vi "Path Edit.vi"() -> ()   [LabVIEW 2019]
uses:
  Classes/Settings/ObjectSettings/ObjectSettings.lvclass/ObjectSettings.ctl
  Classes/Settings/Path Settings/Path Settings.lvclass/Path Settings.ctl
  typedefs/Schedule Types/Schedule--Constant.ctl
  Classes/Settings/Setting Database/Setting Database.lvclass
  Classes/Settings/Path Settings/Path Settings.lvclass
  C:/Users/Albro/Documents/GitHub/AFM-Lithography/lvsrc/Classes/Settings/ObjectSettings/ObjectSettings.lvclass
  Classes/Settings/Setting Database/Typedefs/PrivateEvents--Setting Database.SetDefaultPath.ctl
  <vilib>/JKI/JKI SMO/SMO/SMO.lvclass
  Classes/Settings/Setting Database/Typedefs/PrivateEvents--Setting Database.CopyActivePathToAll.ctl
  Classes/Settings/ObjectSettings/Accessors/Write Voltage Schedule.vi
  Classes/Settings/ObjectSettings/Accessors/Write Speed Schedule.vi
  Classes/Settings/ObjectSettings/Accessors/Write Direction.vi
  Classes/Settings/ObjectSettings/Accessors/Write Resistance.vi
  Classes/Settings/ObjectSettings/Accessors/Write Enabled.vi
  Classes/Settings/Path Settings/Accessors/Write Fill Orientation.vi
  Classes/Settings/Path Settings/Accessors/Write Smooth Segments.vi
  Classes/Settings/ObjectSettings/Accessors/Read Speed Settings.vi
  Classes/Settings/ObjectSettings/Accessors/Read Voltage Settings.vi
  Classes/Settings/Path Settings/Accessors/Write Fill Spacing.vi
  Classes/Settings/Path Settings/Accessors/Write Interpolation.vi
  Classes/Settings/Path Settings/Accessors/Read Interpolation.vi
  Classes/Settings/ObjectSettings/Accessors/Read Enabled.vi
  Classes/Settings/ObjectSettings/Accessors/Read Direction.vi
  Classes/Settings/Path Settings/Accessors/Read Fill Orientation.vi
  Classes/Settings/Path Settings/Accessors/Read Smooth Segments.vi
  Classes/Settings/Path Settings/Accessors/Read Fill Spacing.vi
  Classes/Settings/ObjectSettings/Accessors/Read Speed Schedule.vi
  Classes/Settings/ObjectSettings/Accessors/Read Voltage Schedule.vi
  Classes/Settings/ObjectSettings/Accessors/Read Resistance.vi
  Classes/Settings/ObjectSettings/ObjectSettings.lvclass
panel:
  out "ID String":string
  in  "Apply All":bool
  in  "Apply":bool
  out "Group String":string
  in  "Deviate Settings":bool
  in  "Deviate?":bool=TRUE
  in  "Save Default":bool
  in  "Interpolation":dbl caption="Numeric 2"
  in  "Voltage Settings":bool
  in  "Speed Settings":bool
  in  "Fill Spacing":dbl caption="Numeric 2"
  in  "Fill Orientation":u16(ring) caption="Ring" items=["Horizontal", "Vertical"]
  in  "Smooth Segments":dbl caption="Numeric 2"
  in  "Set Resistance":T1(ring) caption="Enum"
  in  "Copy to All":bool
  in  "Voltage (V)":dbl caption="Numeric 2"
  in  "Speed (um/s)":dbl caption="Numeric 2"
  in  "Voltage Schedule":u16(ring) caption="Ring" items=["Constant", "Ramp", "Fn. Generator", "Formula"]
  in  "Speed Schedule":u16(ring) caption="Ring" items=["Constant", "Ramp", "Fn. Generator", "Formula"]
  in  "Direction":u16(ring) caption="Ring" items=["Forward", "Backward"]
  in  "Enabled?":bool=TRUE
  in  "Index":i32=8
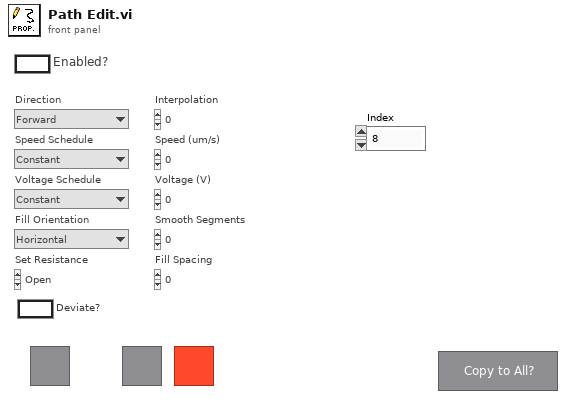
[diagram p1: front panel]
types:
  T1 = enum16{"Open", "Discharge Tip", "0 ohm", "100 kohm", "10 Mohm", "1 Gohm"}
  T2 = typedef "Schedule--Constant.ctl" = cluster{"Value":dbl}
  T3 = enum32{"invalid app kind", "Development System", "Run Time System", "Student Edition", "Embedded LabVIEW", "Evaluation", "Custom"}
  T4 = enum8{"Enabled", "Disabled", "Disabled and Grayed Out"}
  T5 = enum32{"Invalid", "Standard", "Closed", "Hidden", "Minimized", "Maximized"}
  T6 = typedef "Setting Database.lvclass/PrivateEvents--Setting Database.SetDefaultPath.ctl" = bool
  T7 = typedef "Setting Database.lvclass/PrivateEvents--Setting Database.CopyActivePathToAll.ctl" = bool
  T8 = typedef "Setting Database.lvclass/PublicEvents--Setting Database.NewActivePath.ctl" = refnum<class "Path Settings.lvclass">
  T9 = cluster{"Core":cluster{"Current VI Reference":refnum<vi>, "Close Panel on Exit?":bool}, "SettingDB":refnum<class "Setting Database.lvclass">, "Path Settings":refnum<class "Path Settings.lvclass">}
  T10 = cluster{"Current VI Reference":refnum<vi>, "Close Panel on Exit?":bool}
  T11 = typedef "Setting Database.lvclass/PublicEvents--Cluster.ctl" = cluster{"NewActivePath":refnum<user-event>, "PathsUpdated":refnum<user-event>, "RectanglesUpdated":refnum<user-event>, "NewActiveRectangle":refnum<user-event>, "NewActiveFunnel":refnum<user-event>, "FunnelsUpdated":refnum<user-event>, "NewActiveDot":refnum<user-event>, "DotsUpdated":refnum<user-event>}
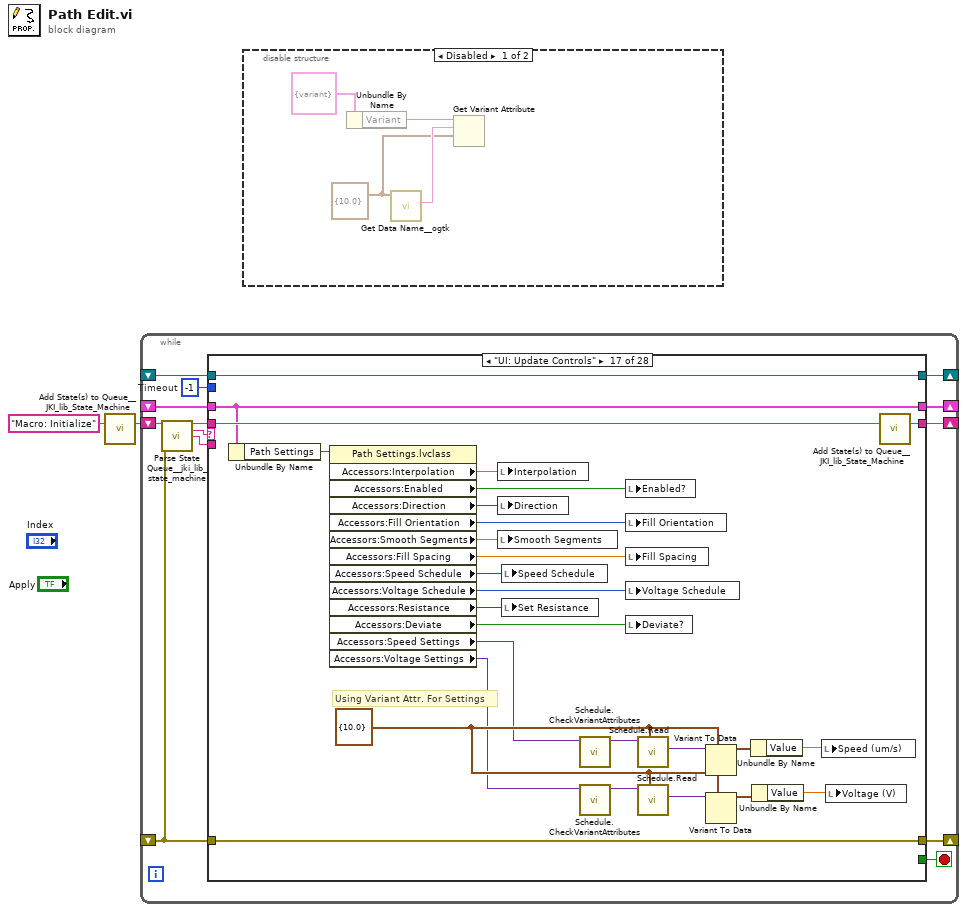
[diagram p0: block diagram]
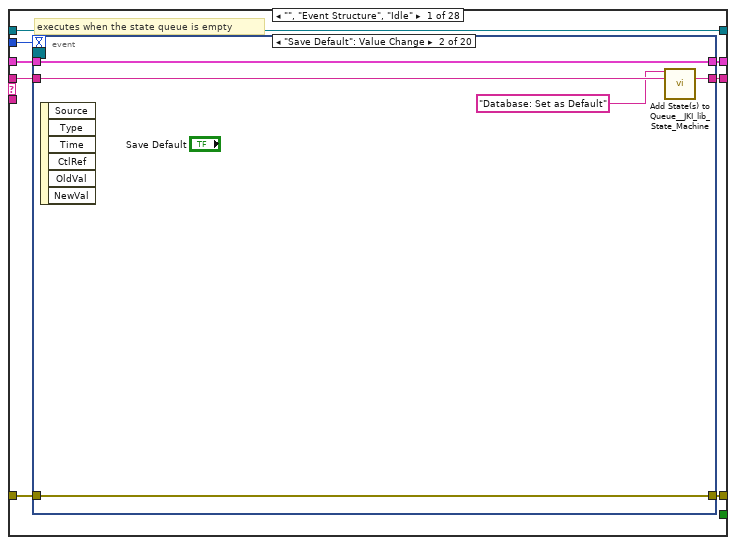
[diagram p3: hidden frame]
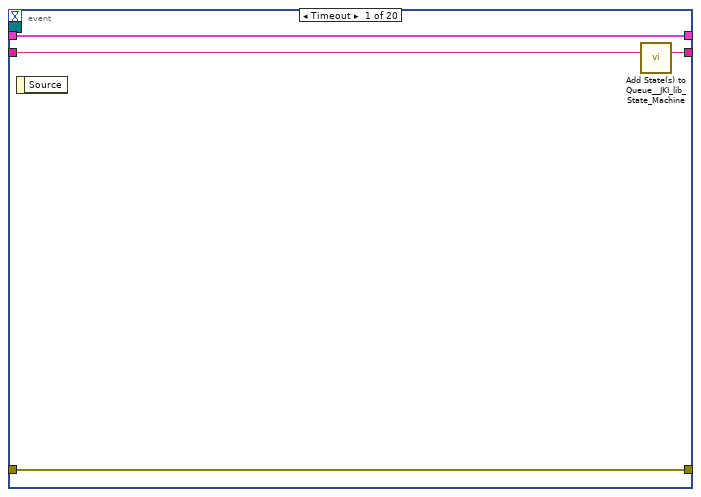
[diagram p4: hidden frame]
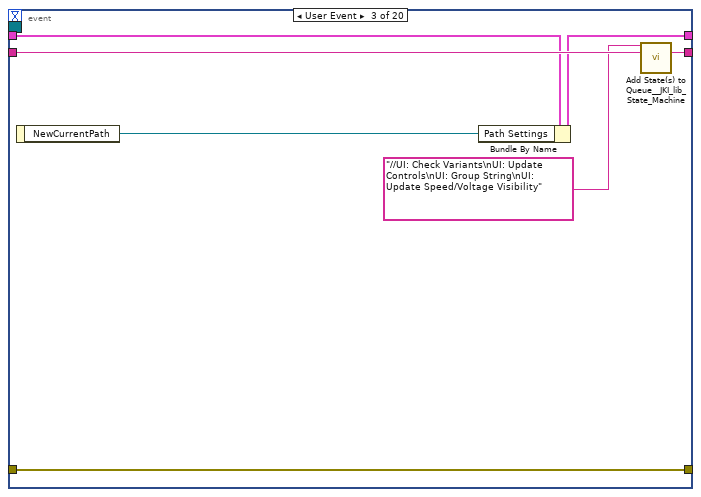
[diagram p5: hidden frame]
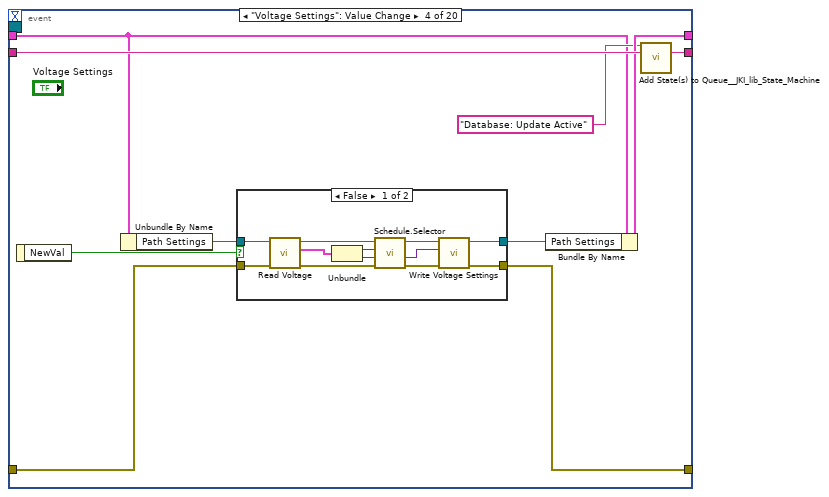
[diagram p6: hidden frame]
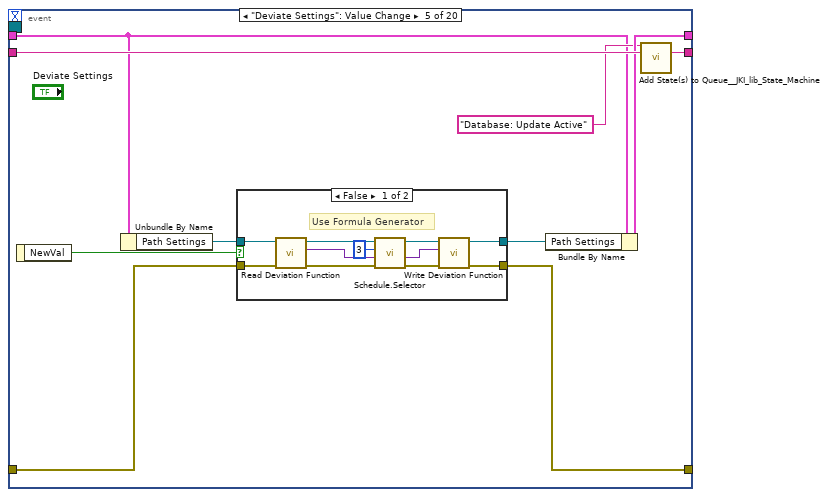
[diagram p8: hidden frame]
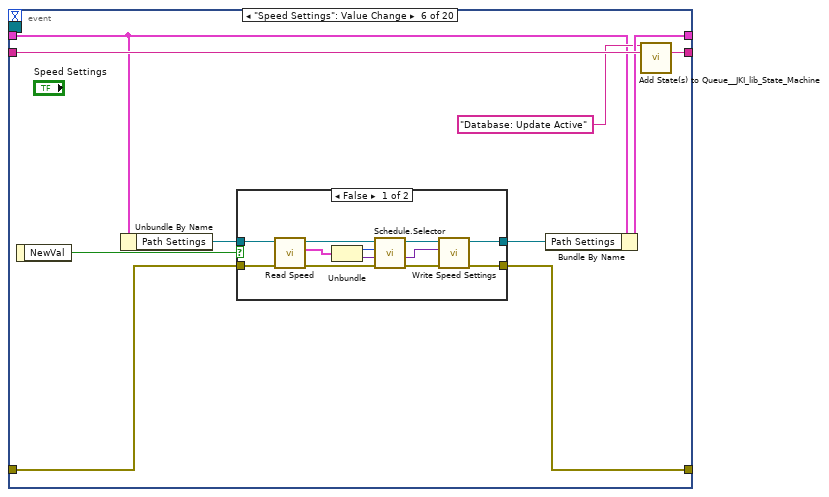
[diagram p10: hidden frame]
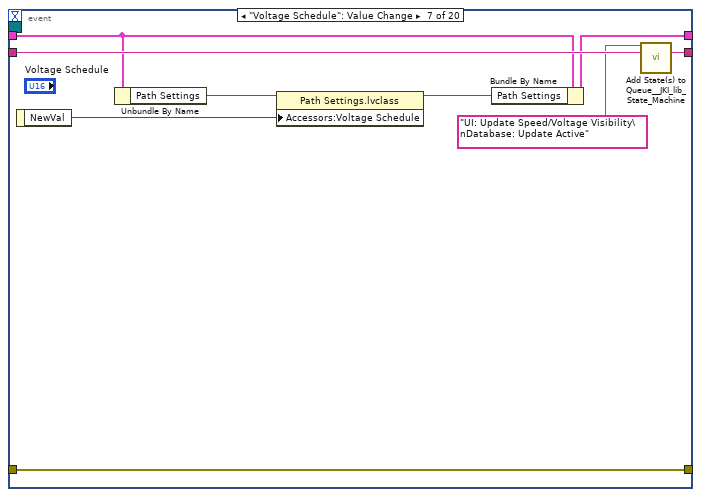
[diagram p12: hidden frame]
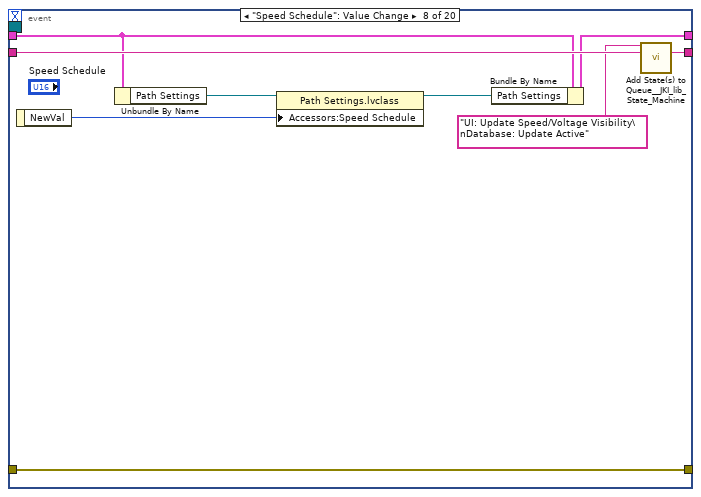
[diagram p13: hidden frame]
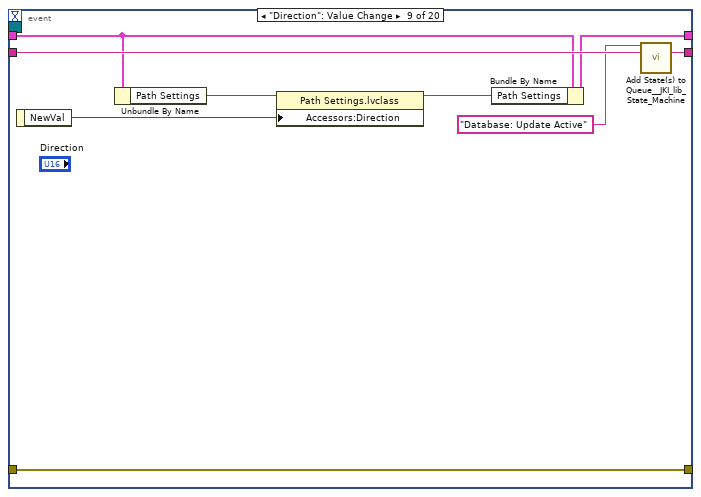
[diagram p14: hidden frame]
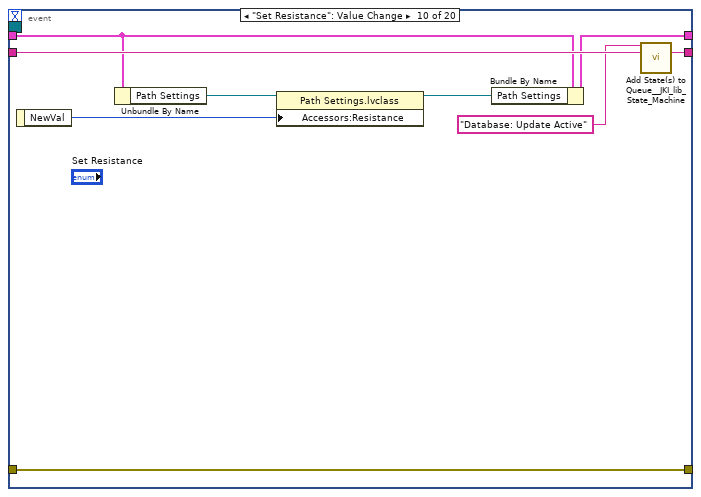
[diagram p15: hidden frame]
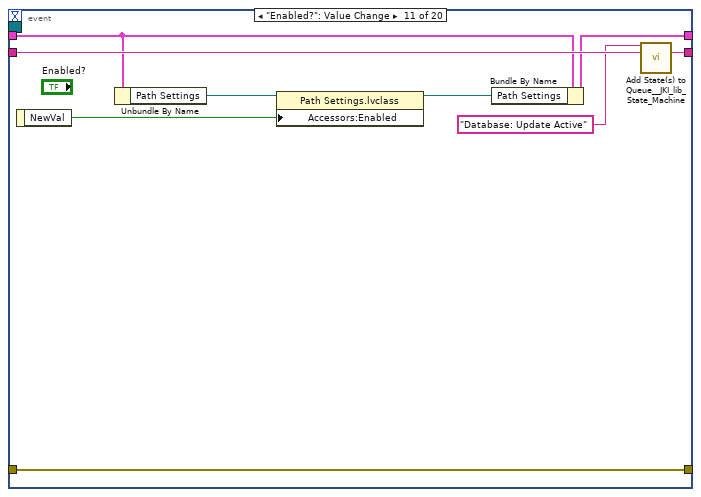
[diagram p16: hidden frame]
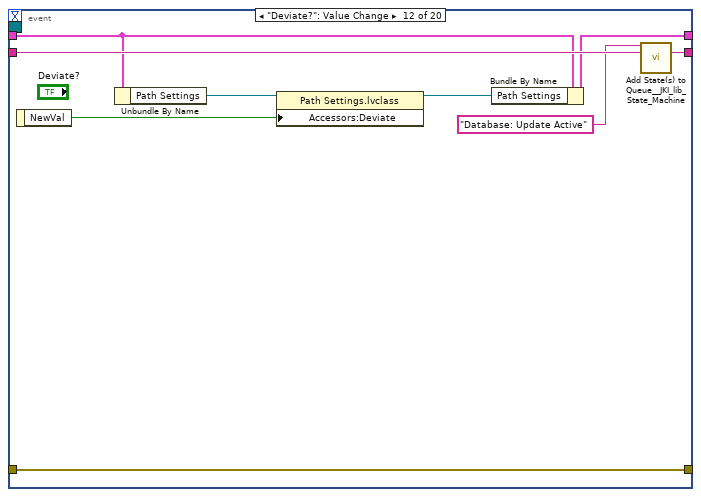
[diagram p17: hidden frame]
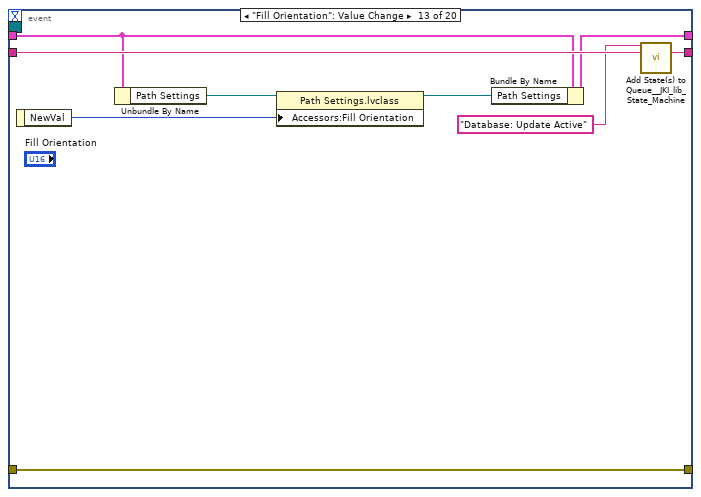
[diagram p18: hidden frame]
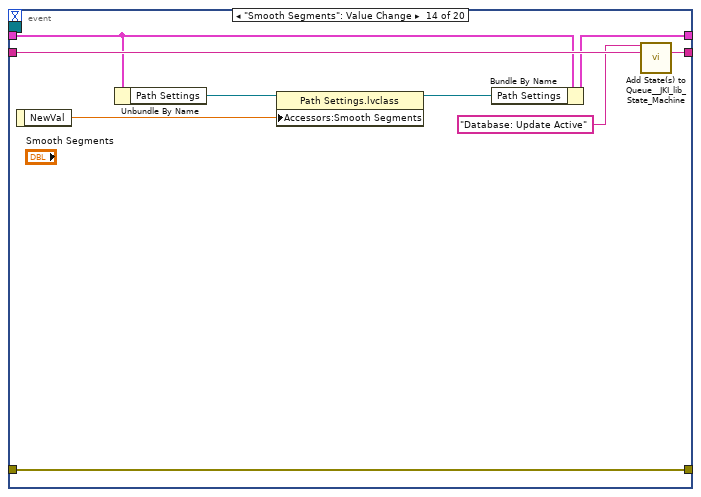
[diagram p19: hidden frame]
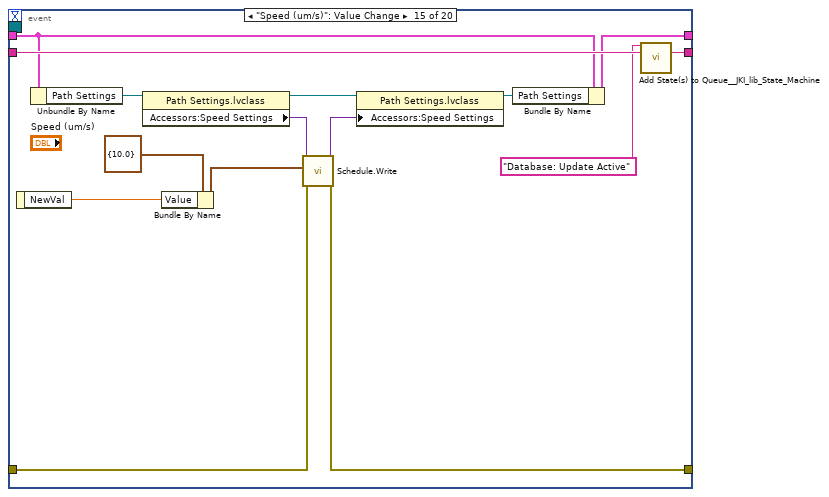
[diagram p20: hidden frame]
diagram:
  n1 = call <vilib>:"Add State(s) to Queue__JKI_lib_State_Machine.vi"("State(s) in (\"\")"="Macro: Initialize") -> ("States Out"=w2:string)  [unwired: 14 in]
  n2 = while "JKI - String-Based Queued State Machine (Basic) v1.0" {
    shift-right: [w8] -> _
    shift-left: _ -> [w6]
    shift-right: [w11] -> _
    shift-left: _ -> [w5]
    shift-right: [w10] -> _
    shift-left: w2 -> [w12]
    shift-right: [w4] -> _
    shift-left: _ -> [w3]
    stop <- w9 stop-if-true
    w7 = -1  # Timeout
    n3 = call <vilib>:"Parse State Queue__jki_lib_state_machine.vi"("State Queue"=w12, "Error In (no error)"=w5) -> ("Remaining States"=w14:string, "Current State"=w15:string, "Arguments"=w13:string)  [unwired: 11 in]
    n4 = case shown="\"UI: Update Controls\"" w15 {
      selector: w15 -> [_ _ w252 _ _ _ _ _ _ _ _ _ _ _ _ _ _ _ _ _ _ _ _ _ _ _ _ _]
      tunnel: w14 -> [w23 w246 w248 w271 w278 w284 w289 w297 w304 w309 w319 w325 w330 w343 w356 w367 w394 w401 w420 w432 w459 w465 w476 w481 w491 w508 w518 w528]
      tunnel: w13 -> [_ _ _ _ _ _ _ _ _ _ _ _ _ _ _ _ _ w397 _ w427 _ _ _ _ _ _ _ _]
      tunnel: [w20 w244 w255 w269 errorcluster {"status"=FALSE, "code"=0, "source"=""} ("error out") w282 w287 w294 w299 w307 w312 w320 w328 w333 w354 w358 w392 w398 w408 w429 w457 w463 w474 w479 w484 w506 w510 w520] -> w11
      tunnel: w5 -> [w19 w244 w254 w269 w275 w282 w287 w294 w300 w307 w310 w321 w328 w339 w354 w361 w392 w399 w416 w430 w457 w463 w474 w479 w483 w506 w509 w519]
      tunnel: [w22 w245 w253 w270 w277 w283 w288 w296 w303 w308 w318 w324 w329 w342 w355 w366 w393 w400 w419 w431 w458 w464 w475 w480 w490 w507 w517 w527] -> w10
      tunnel: [_ _ _ _ _ TRUE _ _ _ _ _ _ _ _ _ _ _ _ _ _ _ _ _ _ _ _ _ _] -> w9
      tunnel: [w18 w243 w251 w262 w273 w280 w286 w293 w301 w306 w316 w323 w327 w340 w352 w365 w388 w396 w418 w426 w456 w461 w468 w478 w488 w498 w515 w525] -> w8
      tunnel: w7 -> [w17 _ _ _ _ _ _ _ _ _ _ _ _ _ _ _ _ _ _ _ _ _ _ _ _ _ _ _]
      tunnel: w6 -> [w21 w243 w251 w263 w273 w280 w286 _ w301 w306 w316 w323 w327 w340 w351 w365 w388 w396 w418 w426 w456 w461 w468 w478 w487 w492 w514 w524]
      tunnel: [w16 w242 w247 w259 w272 w279 w285 w291 w298 w305 w317 w322 w326 w341 w353 w364 w389 w395 w406 w425 w455 w460 w466 w477 w489 w496 w516 w526] -> w4
      tunnel: w3 -> [w16 w242 w247 w259 w272 w279 w285 w291 w298 w305 _ w322 w326 w341 w353 w364 w389 w395 w406 w425 w455 w460 w466 w477 w489 w496 w516 w526]
      frame "", "Event Structure", "Idle" {
        # "executes when the state queue is empty"
        n5 = event shown="[1] \"Save Default\": Value Change" {
          selector: w16 -> [_ _ _ _ _ _ _ _ _ _ _ _ _ _ _ _ _ _ _ _]
          dyn-events: _ -> [_ _ _ _ _ _ _ _ _ _ _ _ _ _ _ _ _ _ _ _]
          timeout: w17 -> [_ _ _ _ _ _ _ _ _ _ _ _ _ _ _ _ _ _ _ _]
          tunnel: w23 -> [w27 w32 w39 w49 w73 w96 w119 w128 w137 w146 w155 w164 w173 w182 w197 w212 w221 w230 w235 w241]
          tunnel: [w26 w31 w38 w48 w72 w95 w118 w127 w136 w145 w154 w163 w172 w181 w196 w211 w220 w229 w234 w240] -> w22
          tunnel: w21 -> [w24 w29 w35 w45 w69 w92 w112 w121 w130 w139 w148 w157 w166 w175 w192 w207 w214 w223 w233 w238]
          tunnel: [w25 w30 w37 w41 w65 w88 w117 w126 w135 w144 w153 w162 w171 w180 w184 w199 w219 w228 w232 w239] -> w20
          tunnel: w19 -> [w25 w30 w37 w40 w64 w87 w117 w126 w135 w144 w153 w162 w171 w180 w183 w198 w219 w228 w232 w239]
          tunnel: [w24 w29 w36 w47 w71 w94 w116 w125 w134 w143 w152 w161 w170 w179 w195 w210 w218 w227 w233 w238] -> w18
          event Timeout {
            n6 = event-data() -> ()  [unwired: 1 in, 1 out]
            n7 = call <vilib>:"Add State(s) to Queue__JKI_lib_State_Machine.vi"("State(s) in (\"\")"=w27) -> ("States Out"=w26:string)  [unwired: 14 in]
          }
          event "Save Default": Value Change {
            n8 = event-data() -> ()  [unwired: 1 in, 6 out]
            n9 = call <vilib>:"Add State(s) to Queue__JKI_lib_State_Machine.vi"("State(s) in Front (\"\")"="Database: Set as Default", "State(s) in (\"\")"=w32) -> ("States Out"=w31:string)  [unwired: 13 in]
          }
          event User Event {
            n10 = event-data() -> ("NewCurrentPath"=w34:T8)  [unwired: 1 in]
            n11 = Bundle By Name(cluster=w35, "Path Settings"=w34) -> (w36:T9)
            n12 = call <vilib>:"Add State(s) to Queue__JKI_lib_State_Machine.vi"("State(s) in Front (\"\")"="//UI: Check Variants\nUI: Update Controls\nUI: Group String\nUI: Update Speed/Voltage Visibility", "State(s) in (\"\")"=w39) -> ("States Out"=w38:string)  [unwired: 13 in]
          }
          event "Voltage Settings": Value Change {
            n13 = event-data() -> ("NewVal"=w44:bool)  [unwired: 1 in]
            n14 = Unbundle By Name(w45) -> ("Path Settings"=w43:refnum<class "Path Settings.lvclass">)
            n15 = case shown="False" w44 {
              tunnel: w43 -> [w61 w63]
              tunnel: [w53 w63] -> w42
              tunnel: w40 -> [w60 w62]
              tunnel: [w50 w62] -> w41
              frame False {
                n16 = call "Read Voltage.vi"("error in (no error)"=w60, "ObjectSettings in"=w61) -> ("error out"=w58:errorcluster, "Voltage"=w57:cluster{"Schedule":u16, "Settings":variant}, "ObjectSettings out"=w59:refnum<class "Path Settings.lvclass">)  [unwired: 7 in]
                n17 = Unbundle(w57) -> ("Schedule"=w56:u16, "Settings"=w55:variant)
                n18 = call-dynamic "Schedule.Selector.vi"("error in (no error)"=w58, "Settings In"=w55, "Schedule"=w56, "ObjectSettings in"=w59) -> ("error out"=w52:errorcluster, "Settings Out"=w51:variant, "ObjectSettings out"=w54:refnum<class "Path Settings.lvclass">)  [unwired: 5 in]
                n19 = call "Write Voltage Settings.vi"("error in (no error)"=w52, "Settings"=w51, "ObjectSettings in"=w54) -> ("error out"=w50:errorcluster, "ObjectSettings out"=w53:refnum<class "Path Settings.lvclass">)  [unwired: 7 in]
              }
              frame True {
              }
            }
            n20 = Bundle By Name(cluster=w45, "Path Settings"=w42) -> (w47:T9)
            n21 = call <vilib>:"Add State(s) to Queue__JKI_lib_State_Machine.vi"("State(s) in Front (\"\")"="Database: Update Active", "State(s) in (\"\")"=w49) -> ("States Out"=w48:string)  [unwired: 13 in]
          }
          event "Deviate Settings": Value Change {
            n22 = event-data() -> ("NewVal"=w68:bool)  [unwired: 1 in]
            n23 = Unbundle By Name(w69) -> ("Path Settings"=w67:refnum<class "Path Settings.lvclass">)
            n24 = case shown="False" w68 {
              tunnel: w67 -> [w79 w86]
              tunnel: [w83 w86] -> w66
              tunnel: w64 -> [w76 w85]
              tunnel: [w80 w85] -> w65
              frame False {
                # "Use Formula Generator"
                n25 = call-dynamic "Read Deviation Function.vi"("error in (no error)"=w76, "Path Settings in"=w79) -> ("error out"=w77:errorcluster, "Deviation Function"=w75:variant, "Path Settings out"=w78:refnum<class "Path Settings.lvclass">)  [unwired: 7 in]
                n26 = call-dynamic "Schedule.Selector.vi"("error in (no error)"=w77, "Settings In"=w75, "Schedule"=u16 3, "ObjectSettings in"=w78) -> ("error out"=w82:errorcluster, "Settings Out"=w81:variant, "ObjectSettings out"=w84:refnum<class "Path Settings.lvclass">)  [unwired: 5 in]
                n27 = call-dynamic "Write Deviation Function.vi"("error in (no error)"=w82, "Deviation Function"=w81, "Path Settings in"=w84) -> ("error out"=w80:errorcluster, "Path Settings out"=w83:refnum<class "Path Settings.lvclass">)  [unwired: 7 in]
              }
              frame True {
              }
            }
            n28 = Bundle By Name(cluster=w69, "Path Settings"=w66) -> (w71:T9)
            n29 = call <vilib>:"Add State(s) to Queue__JKI_lib_State_Machine.vi"("State(s) in Front (\"\")"="Database: Update Active", "State(s) in (\"\")"=w73) -> ("States Out"=w72:string)  [unwired: 13 in]
          }
          event "Speed Settings": Value Change {
            n30 = event-data() -> ("NewVal"=w91:bool)  [unwired: 1 in]
            n31 = Unbundle By Name(w92) -> ("Path Settings"=w90:refnum<class "Path Settings.lvclass">)
            n32 = case shown="False" w91 {
              tunnel: w90 -> [w106 w110]
              tunnel: [w100 w110] -> w89
              tunnel: w87 -> [w104 w109]
              tunnel: [w99 w109] -> w88
              frame False {
                n33 = call "Read Speed.vi"("error in (no error)"=w104, "ObjectSettings in"=w106) -> ("error out"=w103:errorcluster, "Speed"=w102:cluster{"Schedule":u16, "Settings":variant}, "ObjectSettings out"=w105:refnum<class "Path Settings.lvclass">)  [unwired: 7 in]
                n34 = Unbundle(w102) -> ("Schedule"=w108:u16, "Settings"=w107:variant)
                n35 = call-dynamic "Schedule.Selector.vi"("error in (no error)"=w103, "Settings In"=w107, "Schedule"=w108, "ObjectSettings in"=w105) -> ("error out"=w98:errorcluster, "Settings Out"=w97:variant, "ObjectSettings out"=w101:refnum<class "Path Settings.lvclass">)  [unwired: 5 in]
                n36 = call "Write Speed Settings.vi"("error in (no error)"=w98, "Settings"=w97, "ObjectSettings in"=w101) -> ("error out"=w99:errorcluster, "ObjectSettings out"=w100:refnum<class "Path Settings.lvclass">)  [unwired: 7 in]
              }
              frame True {
              }
            }
            n37 = Bundle By Name(cluster=w92, "Path Settings"=w89) -> (w94:T9)
            n38 = call <vilib>:"Add State(s) to Queue__JKI_lib_State_Machine.vi"("State(s) in Front (\"\")"="Database: Update Active", "State(s) in (\"\")"=w96) -> ("States Out"=w95:string)  [unwired: 13 in]
          }
          event "Voltage Schedule": Value Change {
            n39 = event-data() -> ("NewVal"=w111:u16)  [unwired: 1 in]
            n40 = Unbundle By Name(w112) -> ("Path Settings"=w114:refnum<class "Path Settings.lvclass">)
            n41 = property class="Path Settings.lvclass"(reference=w114, "Accessors:Voltage Schedule"=w111) -> (reference out=w113:refnum<class "Path Settings.lvclass">)  [unwired: 1 in, 1 out]
            n42 = Bundle By Name(cluster=w112, "Path Settings"=w113) -> (w116:T9)
            n43 = call <vilib>:"Add State(s) to Queue__JKI_lib_State_Machine.vi"("State(s) in Front (\"\")"="UI: Update Speed/Voltage Visibility\nDatabase: Update Active", "State(s) in (\"\")"=w119) -> ("States Out"=w118:string)  [unwired: 13 in]
          }
          event "Speed Schedule": Value Change {
            n44 = event-data() -> ("NewVal"=w120:u16)  [unwired: 1 in]
            n45 = Unbundle By Name(w121) -> ("Path Settings"=w123:refnum<class "Path Settings.lvclass">)
            n46 = property class="Path Settings.lvclass"(reference=w123, "Accessors:Speed Schedule"=w120) -> (reference out=w122:refnum<class "Path Settings.lvclass">)  [unwired: 1 in, 1 out]
            n47 = Bundle By Name(cluster=w121, "Path Settings"=w122) -> (w125:T9)
            n48 = call <vilib>:"Add State(s) to Queue__JKI_lib_State_Machine.vi"("State(s) in Front (\"\")"="UI: Update Speed/Voltage Visibility\nDatabase: Update Active", "State(s) in (\"\")"=w128) -> ("States Out"=w127:string)  [unwired: 13 in]
          }
          event "Direction": Value Change {
            n49 = event-data() -> ("NewVal"=w129:u16)  [unwired: 1 in]
            n50 = Unbundle By Name(w130) -> ("Path Settings"=w132:refnum<class "Path Settings.lvclass">)
            n51 = property class="Path Settings.lvclass"(reference=w132, "Accessors:Direction"=w129) -> (reference out=w131:refnum<class "Path Settings.lvclass">)  [unwired: 1 in, 1 out]
            n52 = Bundle By Name(cluster=w130, "Path Settings"=w131) -> (w134:T9)
            n53 = call <vilib>:"Add State(s) to Queue__JKI_lib_State_Machine.vi"("State(s) in Front (\"\")"="Database: Update Active", "State(s) in (\"\")"=w137) -> ("States Out"=w136:string)  [unwired: 13 in]
          }
          event "Set Resistance": Value Change {
            n54 = event-data() -> ("NewVal"=w138:T1)  [unwired: 1 in]
            n55 = Unbundle By Name(w139) -> ("Path Settings"=w141:refnum<class "Path Settings.lvclass">)
            n56 = property class="Path Settings.lvclass"(reference=w141, "Accessors:Resistance"=w138) -> (reference out=w140:refnum<class "Path Settings.lvclass">)  [unwired: 1 in, 1 out]
            n57 = Bundle By Name(cluster=w139, "Path Settings"=w140) -> (w143:T9)
            n58 = call <vilib>:"Add State(s) to Queue__JKI_lib_State_Machine.vi"("State(s) in Front (\"\")"="Database: Update Active", "State(s) in (\"\")"=w146) -> ("States Out"=w145:string)  [unwired: 13 in]
          }
          event "Enabled?": Value Change {
            n59 = event-data() -> ("NewVal"=w147:bool)  [unwired: 1 in]
            n60 = Unbundle By Name(w148) -> ("Path Settings"=w150:refnum<class "Path Settings.lvclass">)
            n61 = property class="Path Settings.lvclass"(reference=w150, "Accessors:Enabled"=w147) -> (reference out=w149:refnum<class "Path Settings.lvclass">)  [unwired: 1 in, 1 out]
            n62 = Bundle By Name(cluster=w148, "Path Settings"=w149) -> (w152:T9)
            n63 = call <vilib>:"Add State(s) to Queue__JKI_lib_State_Machine.vi"("State(s) in Front (\"\")"="Database: Update Active", "State(s) in (\"\")"=w155) -> ("States Out"=w154:string)  [unwired: 13 in]
          }
          event "Deviate?": Value Change {
            n64 = event-data() -> ("NewVal"=w156:bool)  [unwired: 1 in]
            n65 = Unbundle By Name(w157) -> ("Path Settings"=w159:refnum<class "Path Settings.lvclass">)
            n66 = property class="Path Settings.lvclass"(reference=w159, "Accessors:Deviate"=w156) -> (reference out=w158:refnum<class "Path Settings.lvclass">)  [unwired: 1 in, 1 out]
            n67 = Bundle By Name(cluster=w157, "Path Settings"=w158) -> (w161:T9)
            n68 = call <vilib>:"Add State(s) to Queue__JKI_lib_State_Machine.vi"("State(s) in Front (\"\")"="Database: Update Active", "State(s) in (\"\")"=w164) -> ("States Out"=w163:string)  [unwired: 13 in]
          }
          event "Fill Orientation": Value Change {
            n69 = event-data() -> ("NewVal"=w165:u16)  [unwired: 1 in]
            n70 = Unbundle By Name(w166) -> ("Path Settings"=w168:refnum<class "Path Settings.lvclass">)
            n71 = property class="Path Settings.lvclass"(reference=w168, "Accessors:Fill Orientation"=w165) -> (reference out=w167:refnum<class "Path Settings.lvclass">)  [unwired: 1 in, 1 out]
            n72 = Bundle By Name(cluster=w166, "Path Settings"=w167) -> (w170:T9)
            n73 = call <vilib>:"Add State(s) to Queue__JKI_lib_State_Machine.vi"("State(s) in Front (\"\")"="Database: Update Active", "State(s) in (\"\")"=w173) -> ("States Out"=w172:string)  [unwired: 13 in]
          }
          event "Smooth Segments": Value Change {
            n74 = event-data() -> ("NewVal"=w174:dbl)  [unwired: 1 in]
            n75 = Unbundle By Name(w175) -> ("Path Settings"=w177:refnum<class "Path Settings.lvclass">)
            n76 = property class="Path Settings.lvclass"(reference=w177, "Accessors:Smooth Segments"=w174) -> (reference out=w176:refnum<class "Path Settings.lvclass">)  [unwired: 1 in, 1 out]
            n77 = Bundle By Name(cluster=w175, "Path Settings"=w176) -> (w179:T9)
            n78 = call <vilib>:"Add State(s) to Queue__JKI_lib_State_Machine.vi"("State(s) in Front (\"\")"="Database: Update Active", "State(s) in (\"\")"=w182) -> ("States Out"=w181:string)  [unwired: 13 in]
          }
          event "Speed (um/s)": Value Change {
            n79 = event-data() -> ("NewVal"=w190:dbl)  [unwired: 1 in]
            n80 = Unbundle By Name(w192) -> ("Path Settings"=w189:refnum<class "Path Settings.lvclass">)
            n81 = property class="Path Settings.lvclass"(reference=w189) -> (reference out=w188:refnum<class "Path Settings.lvclass">, "Accessors:Speed Settings"=w187:variant)  [unwired: 1 in, 1 out]
            n82 = Bundle By Name(cluster=T2 {"Value"=10.0} ("Constant"), "Value"=w190) -> (w185:T2)
            n83 = call "Schedule.Write.vi"("error in (no error)"=w183, "Data to Write"=w185, "LUT In"=w187) -> ("error out"=w184:errorcluster, "LUT Out"=w186:variant)  [unwired: 7 in]
            n84 = property class="Path Settings.lvclass"(reference=w188, "Accessors:Speed Settings"=w186) -> (reference out=w193:refnum<class "Path Settings.lvclass">)  [unwired: 1 in, 1 out]
            n85 = Bundle By Name(cluster=w192, "Path Settings"=w193) -> (w195:T9)
            n86 = call <vilib>:"Add State(s) to Queue__JKI_lib_State_Machine.vi"("State(s) in Front (\"\")"="Database: Update Active", "State(s) in (\"\")"=w197) -> ("States Out"=w196:string)  [unwired: 13 in]
          }
          event "Voltage (V)": Value Change {
            n87 = event-data() -> ("NewVal"=w205:dbl)  [unwired: 1 in]
            n88 = Unbundle By Name(w207) -> ("Path Settings"=w204:refnum<class "Path Settings.lvclass">)
            n89 = property class="Path Settings.lvclass"(reference=w204) -> (reference out=w203:refnum<class "Path Settings.lvclass">, "Accessors:Voltage Settings"=w202:variant)  [unwired: 1 in, 1 out]
            n90 = Bundle By Name(cluster=T2 {"Value"=10.0} ("Constant"), "Value"=w205) -> (w200:T2)
            n91 = call "Schedule.Write.vi"("error in (no error)"=w198, "Data to Write"=w200, "LUT In"=w202) -> ("error out"=w199:errorcluster, "LUT Out"=w201:variant)  [unwired: 7 in]
            n92 = property class="Path Settings.lvclass"(reference=w203, "Accessors:Voltage Settings"=w201) -> (reference out=w208:refnum<class "Path Settings.lvclass">)  [unwired: 1 in, 1 out]
            n93 = Bundle By Name(cluster=w207, "Path Settings"=w208) -> (w210:T9)
            n94 = call <vilib>:"Add State(s) to Queue__JKI_lib_State_Machine.vi"("State(s) in Front (\"\")"="Database: Update Active", "State(s) in (\"\")"=w212) -> ("States Out"=w211:string)  [unwired: 13 in]
          }
          event "Fill Spacing": Value Change {
            n95 = event-data() -> ("NewVal"=w213:dbl)  [unwired: 1 in]
            n96 = Unbundle By Name(w214) -> ("Path Settings"=w216:refnum<class "Path Settings.lvclass">)
            n97 = property class="Path Settings.lvclass"(reference=w216, "Accessors:Fill Spacing"=w213) -> (reference out=w215:refnum<class "Path Settings.lvclass">)  [unwired: 1 in, 1 out]
            n98 = Bundle By Name(cluster=w214, "Path Settings"=w215) -> (w218:T9)
            n99 = call <vilib>:"Add State(s) to Queue__JKI_lib_State_Machine.vi"("State(s) in Front (\"\")"="Database: Update Active", "State(s) in (\"\")"=w221) -> ("States Out"=w220:string)  [unwired: 13 in]
          }
          event "Interpolation": Value Change {
            n100 = event-data() -> ("NewVal"=w222:dbl)  [unwired: 1 in]
            n101 = Unbundle By Name(w223) -> ("Path Settings"=w225:refnum<class "Path Settings.lvclass">)
            n102 = property class="Path Settings.lvclass"(reference=w225, "Accessors:Interpolation"=w222) -> (reference out=w224:refnum<class "Path Settings.lvclass">)  [unwired: 1 in, 1 out]
            n103 = Bundle By Name(cluster=w223, "Path Settings"=w224) -> (w227:T9)
            n104 = call <vilib>:"Add State(s) to Queue__JKI_lib_State_Machine.vi"("State(s) in Front (\"\")"="Database: Update Active", "State(s) in (\"\")"=w230) -> ("States Out"=w229:string)  [unwired: 13 in]
          }
          event "Copy to All", "Apply All": Value Change {
            n105 = event-data() -> ()  [unwired: 1 in, 1 out]
            n106 = call <vilib>:"Add State(s) to Queue__JKI_lib_State_Machine.vi"("State(s) in Front (\"\")"="Database: Copy to All", "State(s) in (\"\")"=w235) -> ("States Out"=w234:string)  [unwired: 13 in]
          }
          event Panel Close? {
            # "Discard the event because we'll close the front panel ourselves in Macro: Exit"
            # "Close Panel button (pressed) Event\n(this executes Macro: Exit to terminate the VI)"
            n107 = event-data() -> ()  [unwired: 1 in, 1 out]
            n108 = event-data("Discard?"=TRUE) -> ()  [unwired: 1 in, 1 out]
            n109 = call <vilib>:"Add State(s) to Queue__JKI_lib_State_Machine.vi"("State(s) in Front (\"\")"="Macro: Exit", "State(s) in (\"\")"=w241) -> ("States Out"=w240:string)  [unwired: 13 in]
          }
        }
      }
      frame "---------- Core ----------" {
        # "Do not put any code in this frame.\n(it is a separator no-op)"
        n110 = call <vilib>:"Add State(s) to Queue__JKI_lib_State_Machine.vi"("State(s) in (\"\")"=w246) -> ("States Out"=w245:string)  [unwired: 14 in]
      }
      frame Default {
        w258 = 42 items=["No error", "Argument error", "Memory is full", "Out of zone", "End of file", "File already open", "Generic file I/O error", "File not found", "File permission error", "Disk is full", "Duplicate path", "Too many files open", "System feature not enabled", "Resource file not found", "Cannot add resource", "Resource not found", "Image not found", "Image memory error", "Pen does not exist", "Config type invalid", "Config token not found", "Config parse error", "Config memory error", "Bad external code format", "Bad external code offset", "External code not present", "Null window", "Destroy window error", "Null menu", "Print aborted", "Bad print record", "Print driver error", "Windows error during printing", "Memory error during printing", "Print dialog error", "Generic print error", "Invalid device refnum", "Device not found", "Device parameter error", "Device unit error", "Cannot open device", "Device call aborted", "Generic error", "Cancelled by user", "Object ID too low", "Object ID too high", "Object not in heap", "Unknown heap", "Unknown object (invalid DefProc)", "Unknown object (DefProc not in table)", "Message out of range", "Invalid (null) method", "Unknown message", "Manager call not supported", "Bad address", "Network operation in progress", "Network operation timed out", "Connection is busy", "Network attribute not supported", "Network error", "Address in use", "System out of memory", "Connection aborted", "Connection refused", "Not connected", "Already connected", "Connection closed", "Initialization error (interapplication manager)", "Bad occurrence", "Wait on unbound occurrence handler", "Occurrence queue overflow", "Datalog type conflict", "Unused", "Unrecognized type (interapplication manager)", "Memory corrupt", "Failed to make temporary DLL", "Old CIN version", "Drag socket not found", "Failed to load drop-object", "Failed to register OLE object", "Failed to release OLE object", "Format specifier type mismatch", "Unknown format specifier", "Too few format specifiers", "Too many format specifiers", "Scan failed", "Newer CIN version", "Error converting to variant", "Runtime menu error", "Password tampered", "Variant attribute not found", "Incompatible variant data type", "Event data is not available", "Event Store is not present", "Occurrence is not found", "Event Queue is not created", "Event info is not available", "Refnum passed is NULL", "Error retrieving Class GUID", "Error retrieving CoClass GUID", "Error retrieving TypeLib GUID.", "Bad built application magic bytes.", "Specific driver is different from the specific driver associated with the Logical Name.", "There is no session opened to the class driver.", "Max Error", "MAX - Error with config objects", "MAX - Error loading configuration", "MAX - Group not supported"]
        # "Current State"
        # "Do not delete, rename, or modify this frame.\n(this is used to capture unhandled states and typos)"
        # "Handle mistyped state name (developer tool)"
        n111 = Format Into String(format string="Software Exception: Unhandled State \"%s\"." ("message"), error in=w254, w252) -> (resulting string=w257:string, error out=w256:errorcluster)  [unwired: 1 in]
        n112 = call <vilib>:"Error Cluster From Error Code.vi"("show call chain? (False)"=TRUE, "error in (no error)"=w256, "error message (\"\")"=w257, "error code (0)"=w258) -> ("error out"=w255:errorcluster)  [unwired: 5 in]
        n113 = call <vilib>:"Add State(s) to Queue__JKI_lib_State_Machine.vi"("State(s) in (\"\")"=w248) -> ("States Out"=w253:string)  [unwired: 14 in]
      }
      frame "Initialize Core Data" {
        # "exe?"
        # "If panel starts closed or is an EXE, then close it when we exit"
        # "Do not delete, rename, or modify this frame.\n(this is used to determine panel behavior on exit)"
        n114 = control-ref of="Current VI Reference"() -> (w268:refnum<vi>)
        n115 = property class="VI"() -> ("Front Panel.Open"=w267:bool)  [unwired: 2 in, 2 out]
        n116 = property class="App"() -> ("App.Kind"=w266:T3)  [unwired: 2 in, 2 out]
        n117 = Not(x=w267) -> (.not. x?=w261:bool)
        n118 = Equal?(x=w266, y=T3."Run Time System" ("Application:Kind")) -> (x = y?=w260:bool)
        n119 = Or(x=w261, y=w260) -> (x .or. y?=w264:bool)
        n120 = Bundle By Name(cluster=w263, "Core.Current VI Reference"=w268, "Core.Close Panel on Exit?"=w264) -> (w262:T9)
        n121 = call <vilib>:"Add State(s) to Queue__JKI_lib_State_Machine.vi"("State(s) in (\"\")"=w271) -> ("States Out"=w270:string)  [unwired: 14 in]
      }
      frame "Error Handler" {
        # "Unhandled Error -- Display it"
        # "Handle any errors here.\nYou can also output any states to clean-up after errors occur"
        # "Clear error"
        n122 = call <vilib>:"General Error Handler.vi"("error in (no error)"=w275) -> ()  [unwired: 10 in, 5 out]
        n123 = call <vilib>:"Add State(s) to Queue__JKI_lib_State_Machine.vi"("State(s) in Front (\"\")"="/* Post Error States", "State(s) in (\"\")"=w278) -> ("States Out"=w277:string)  [unwired: 13 in]
      }
      frame "Exit" {
        # "Do not put any code in this frame.\n(No errors that occur here will be handled.)"
        n124 = call <vilib>:"Add State(s) to Queue__JKI_lib_State_Machine.vi"("State(s) in (\"\")"=w284) -> ("States Out"=w283:string)  [unwired: 14 in]
      }
      frame "---------- Data ----------" {
        # "Do not put any code in this frame.\n(It is a separator no-op. You can make a copy of this frame to create a new Data frame)"
        n125 = call <vilib>:"Add State(s) to Queue__JKI_lib_State_Machine.vi"("State(s) in (\"\")"=w289) -> ("States Out"=w288:string)  [unwired: 14 in]
      }
      frame "Data: Initialize" {
        w290 = refnum<class "Path Settings.lvclass"> refnum  # Path Settings
        w292 = refnum<class "Setting Database.lvclass"> refnum  # SettingDB
        w295 = T10 {"Current VI Reference"=refnum, "Close Panel on Exit?"=FALSE}  # Core
        # "Initialize the shift-register data, here.\n(data names are defined by what you wire into the bundle function)"
        n126 = Bundle("Core"=w295, "SettingDB"=w292, "Path Settings"=w290) -> (w293:T9)  [unwired: 1 in]
        n127 = call <vilib>:"Add State(s) to Queue__JKI_lib_State_Machine.vi"("State(s) in (\"\")"=w297) -> ("States Out"=w296:string)  [unwired: 14 in]
      }
      frame "Data: Cleanup" {
        # "Cleanup any data and references, here.\n(this is called automatically, by the Macro: Exit)"
        n128 = Unbundle By Name(w301) -> ("Core.Current VI Reference"=w302:refnum<vi>)
        n129 = Close Reference(reference=w302, error in (no error)=w300) -> (error out=w299:errorcluster)
        n130 = call <vilib>:"Add State(s) to Queue__JKI_lib_State_Machine.vi"("State(s) in (\"\")"=w304) -> ("States Out"=w303:string)  [unwired: 14 in]
      }
      frame "---------- Events ----------" {
        # "Do not put any code in this frame.\n(It is a separator no-op. You can make a copy of this frame to create a new UI frame)"
        n131 = call <vilib>:"Add State(s) to Queue__JKI_lib_State_Machine.vi"("State(s) in (\"\")"=w309) -> ("States Out"=w308:string)  [unwired: 14 in]
      }
      frame "Events: Register" {
        # "Do not put any code in this frame.\n(It is a separator no-op. You can make a copy of this frame to create a new UI frame)"
        n132 = Unbundle By Name(w316) -> ("SettingDB"=w315:refnum<class "Setting Database.lvclass">)
        n133 = call "Setting Database.GetPublicEvents.vi"("Setting Database"=w315) -> ("error out"=w311:errorcluster, "Public Events"=w314:T11)  [unwired: 8 in, 1 out]
        n134 = register-events(w314) -> (reference out=w317:refnum<event-registration>, error out=w313:errorcluster)  [unwired: 2 in]
        n135 = Merge Errors(w310, w313, w311) -> (w312:errorcluster)
        n136 = call <vilib>:"Add State(s) to Queue__JKI_lib_State_Machine.vi"("State(s) in (\"\")"=w319) -> ("States Out"=w318:string)  [unwired: 14 in]
      }
      frame "Events: Unregister" {
        # "Do not put any code in this frame.\n(It is a separator no-op. You can make a copy of this frame to create a new UI frame)"
        n137 = Unregister For Events(event registration refnum=w322, error in=w321) -> (error out=w320:errorcluster)
        n138 = call <vilib>:"Add State(s) to Queue__JKI_lib_State_Machine.vi"("State(s) in (\"\")"=w325) -> ("States Out"=w324:string)  [unwired: 14 in]
      }
      frame "---------- UI ----------" {
        # "Do not put any code in this frame.\n(It is a separator no-op. You can make a copy of this frame to create a new UI frame)"
        n139 = call <vilib>:"Add State(s) to Queue__JKI_lib_State_Machine.vi"("State(s) in (\"\")"=w330) -> ("States Out"=w329:string)  [unwired: 14 in]
      }
      frame "UI: Group String" {
        # "Do not put any code in this frame.\n(It is a separator no-op. You can make a copy of this frame to create a new UI frame)"
        n140 = Unbundle By Name(w340) -> ("Path Settings"=w332:refnum<class "Path Settings.lvclass">)
        n141 = control-ref of="Apply"() -> (w338:refnum<vi>)
        n142 = call-dynamic "Read GUID.vi"("ObjectSettings in"=w332) -> ("GUID"=→"ID String":string)  [unwired: 8 in, 2 out]
        n143 = call-dynamic "Read Group.vi"("error in (no error)"=w339, "ObjectSettings in"=w332) -> ("error out"=w334:errorcluster, "Group"=w337:string)  [unwired: 7 in, 1 out]
        "Group String" <- w337
        n144 = Empty String/Path?(string/path=w337) -> (empty?=w336:bool)
        n145 = Not(x=w336) -> (.not. x?=w335:bool)
        n146 = property class="Bool"(reference=w338, error in=w334, "Visible"=w335) -> (error out=w333:errorcluster)  [unwired: 1 out]
        n147 = call <vilib>:"Add State(s) to Queue__JKI_lib_State_Machine.vi"("State(s) in (\"\")"=w343) -> ("States Out"=w342:string)  [unwired: 14 in]
      }
      frame "UI: Check Variants" {
        # "Do not put any code in this frame.\n(It is a separator no-op. You can make a copy of this frame to create a new UI frame)"
        n148 = Unbundle By Name(w351) -> ("Path Settings"=w350:refnum<class "Path Settings.lvclass">)
        n149 = property class="Path Settings.lvclass"(reference=w350) -> (reference out=w349:refnum<class "Path Settings.lvclass">, "Accessors:Speed Settings"=w347:variant, "Accessors:Voltage Settings"=w345:variant)  [unwired: 1 in, 1 out]
        n150 = call "Schedule.CheckVariantAttributes.vi"("Variant In"=w347) -> ("Variant Out"=w346:variant)  [unwired: 9 in, 1 out]
        n151 = call "Schedule.CheckVariantAttributes.vi"("Variant In"=w345) -> ("Variant Out"=w344:variant)  [unwired: 9 in, 1 out]
        n152 = property class="Path Settings.lvclass"(reference=w349, "Accessors:Speed Settings"=w346, "Accessors:Voltage Settings"=w344) -> (reference out=w348:refnum<class "Path Settings.lvclass">)  [unwired: 1 in, 1 out]
        n153 = Bundle By Name(cluster=w351, "Path Settings"=w348) -> (w352:T9)
        n154 = call <vilib>:"Add State(s) to Queue__JKI_lib_State_Machine.vi"("State(s) in (\"\")"=w356) -> ("States Out"=w355:string)  [unwired: 14 in]
      }
      frame "UI: Initialize" {
        # "Initialize the User Interface, here.\n(this is called automatically, by the Macro: Init)"
        n155 = control-ref of="Speed Schedule"() -> (w363:refnum<vi>)
        n156 = property class="Ring (strict)"(reference=w363, error in=w361, "DisabledEnum"=T4."Disabled and Grayed Out" ("Disabled")) -> (error out=w359:errorcluster)  [unwired: 1 out]
        n157 = control-ref of="Apply All"() -> (w357:refnum<vi>)
        n158 = property class="Bool"(reference=w357, error in=w359, "Colors [4]"=cluster{u32, u32}[] [{16730410, 16730410}, {16730410, 16730410}, {16730410, 16730410}, {16730410, 16730410}]) -> (error out=w358:errorcluster)  [unwired: 1 out]
        n159 = call <vilib>:"Add State(s) to Queue__JKI_lib_State_Machine.vi"("State(s) in (\"\")"=w367) -> ("States Out"=w366:string)  [unwired: 14 in]
      }
      frame "UI: Update Controls" {
        w373 = T2 {"Value"=10.0} ("Constant")
        # "Using Variant Attr. For Settings"
        n160 = Unbundle By Name(w388) -> ("Path Settings"=w387:refnum<class "Path Settings.lvclass">)
        n161 = property class="Path Settings.lvclass"(reference=w387) -> ("Accessors:Interpolation"=w386:dbl, "Accessors:Enabled"=w385:bool, "Accessors:Direction"=w384:u16, "Accessors:Fill Orientation"=w383:u16, "Accessors:Smooth Segments"=w381:dbl, "Accessors:Fill Spacing"=w380:dbl, "Accessors:Speed Schedule"=w382:u16, "Accessors:Voltage Schedule"=w379:u16, "Accessors:Resistance"=w378:T1, "Accessors:Deviate"=w368:bool, "Accessors:Speed Settings"=w372:variant, "Accessors:Voltage Settings"=w370:variant)  [unwired: 1 in, 2 out]
        n162 = local write "Interpolation"(w386) -> ()
        n163 = local write "Direction"(w384) -> ()
        n164 = local write "Smooth Segments"(w381) -> ()
        n165 = local write "Speed Schedule"(w382) -> ()
        n166 = local write "Set Resistance"(w378) -> ()
        n167 = call "Schedule.CheckVariantAttributes.vi"("Variant In"=w372) -> ("Variant Out"=w371:variant)  [unwired: 9 in, 1 out]
        n168 = call "Schedule.CheckVariantAttributes.vi"("Variant In"=w370) -> ("Variant Out"=w369:variant)  [unwired: 9 in, 1 out]
        n169 = local write "Enabled?"(w385) -> ()
        n170 = local write "Fill Orientation"(w383) -> ()
        n171 = local write "Fill Spacing"(w380) -> ()
        n172 = local write "Voltage Schedule"(w379) -> ()
        n173 = local write "Deviate?"(w368) -> ()
        n174 = call "Schedule.Read.vi"("Data to Read"=w373, "LUT In"=w371) -> ("Data Out"=w377:variant)  [unwired: 7 in, 2 out]
        n175 = call "Schedule.Read.vi"("Data to Read"=w373, "LUT In"=w369) -> ("Data Out"=w375:variant)  [unwired: 7 in, 2 out]
        n176 = Variant To Data(type=w373, Variant=w377) -> (data=w376:T2)  [unwired: 1 in, 1 out]
        n177 = Variant To Data(type=w373, Variant=w375) -> (data=w374:T2)  [unwired: 1 in, 1 out]
        n178 = Unbundle By Name(w376) -> ("Value"=w391:dbl)
        n179 = Unbundle By Name(w374) -> ("Value"=w390:dbl)
        n180 = local write "Speed (um/s)"(w391) -> ()
        n181 = local write "Voltage (V)"(w390) -> ()
        n182 = call <vilib>:"Add State(s) to Queue__JKI_lib_State_Machine.vi"("State(s) in (\"\")"=w394) -> ("States Out"=w393:string)  [unwired: 14 in]
      }
      frame "UI: Cursor Set" {
        # "Argument"
        # "Set and Unset Cursor Busy.\n(Usage: \"UI: Cursor Set >> Busy|Idle\")"
        n183 = case shown="\"Idle\", Default" w397 {
          tunnel: w399 -> [w403 w405]
          tunnel: [w402 w404] -> w398
          frame "Idle", Default {
            n184 = call <vilib>:"Unset Busy.vi"("error in (no error)"=w403) -> ("error out"=w402:errorcluster)  [unwired: 10 in]
          }
          frame "Busy" {
            n185 = call <vilib>:"Set Busy.vi"("error in (no error)"=w405) -> ("error out"=w404:errorcluster)  [unwired: 9 in, 1 out]
          }
        }
        n186 = call <vilib>:"Add State(s) to Queue__JKI_lib_State_Machine.vi"("State(s) in (\"\")"=w401) -> ("States Out"=w400:string)  [unwired: 14 in]
      }
      frame "UI: Update Speed/Voltage Visibility" {
        n187 = local read "Voltage Schedule"() -> (w414:u16)
        n188 = local read "Speed Schedule"() -> (w413:u16)
        n189 = case shown="1, Default" w414 {
          tunnel: [TRUE FALSE] -> w417
          frame 0 {
          }
          frame 1, Default {
          }
        }
        n190 = case shown="1, Default" w413 {
          tunnel: [TRUE FALSE] -> w415
          frame 0 {
          }
          frame 1, Default {
          }
        }
        n191 = property on="Voltage (V)" class="DigNum (strict)"(error in=w416, "Visible"=w417) -> (error out=w412:errorcluster)  [unwired: 1 in, 1 out]
        n192 = Not(x=w417) -> (.not. x?=w411:bool)
        n193 = property on="Voltage Settings" class="Bool (strict)"(error in=w412, "Visible"=w411) -> (error out=w410:errorcluster)  [unwired: 1 in, 1 out]
        n194 = property on="Speed (um/s)" class="DigNum (strict)"(error in=w410, "Visible"=w415) -> (error out=w409:errorcluster)  [unwired: 1 in, 1 out]
        n195 = Not(x=w415) -> (.not. x?=w407:bool)
        n196 = property on="Speed Settings" class="Bool (strict)"(error in=w409, "Visible"=w407) -> (error out=w408:errorcluster)  [unwired: 1 in, 1 out]
        n197 = call <vilib>:"Add State(s) to Queue__JKI_lib_State_Machine.vi"("State(s) in (\"\")"=w420) -> ("States Out"=w419:string)  [unwired: 14 in]
      }
      frame "UI: Front Panel State" {
        # "Argument"
        # "Set Front Panel Open or Closed\n(Usage: \"UI: Front Panel State >> Open|Close\")"
        n198 = Unbundle By Name(w426) -> ("Core.Current VI Reference"=w428:refnum<vi>)
        n199 = case shown="\"Open\", Default" w427 {
          tunnel: w430 -> [w436 w449]
          tunnel: [w438 w450] -> w429
          tunnel: w428 -> [w437 w447]
          frame "Open", Default {
            n200 = property class="VI"(reference=w437, error in=w436) -> (reference out=w434:refnum<vi>, error out=w435:errorcluster, "Front Panel.Open"=w433:bool)
            n201 = case shown="False" w433 {
              tunnel: [w441 w444] -> w438
              tunnel: w435 -> [w440 w444]
              tunnel: w434 -> [w439 _]
              frame False {
                n202 = invoke class="VI" method="FP.Open"(reference=w439, error in=w440, "Activate"=TRUE, "State"=T5."Standard") -> (error out=w441:errorcluster)  [unwired: 1 in, 4 out]
              }
              frame True {
              }
            }
          }
          frame "Close" {
            n203 = property class="VI"(reference=w447, error in=w449) -> (reference out=w446:refnum<vi>, error out=w448:errorcluster, "Front Panel.Open"=w445:bool)
            n204 = case shown="True" w445 {
              tunnel: [w451 w454] -> w450
              tunnel: w448 -> [w451 w453]
              tunnel: w446 -> [_ w452]
              frame False {
              }
              frame True {
                n205 = invoke class="VI" method="FP.Close"(reference=w452, error in=w453) -> (error out=w454:errorcluster)  [unwired: 1 in, 2 out]
              }
            }
          }
        }
        n206 = call <vilib>:"Add State(s) to Queue__JKI_lib_State_Machine.vi"("State(s) in (\"\")"=w432) -> ("States Out"=w431:string)  [unwired: 14 in]
      }
      frame "---------- Macro ----------" {
        # "Do not put any code in this frame.\n(It is a separator no-op. You can make a copy of this frame to create a new Macro frame)"
        n207 = call <vilib>:"Add State(s) to Queue__JKI_lib_State_Machine.vi"("State(s) in (\"\")"=w459) -> ("States Out"=w458:string)  [unwired: 14 in]
      }
      frame "Macro: Initialize" {
        # "Initialization Macro\n(This is called once, when the VI starts)"
        n208 = call <vilib>:"Add State(s) to Queue__JKI_lib_State_Machine.vi"("State(s) in Front (\"\")"="Data: Initialize\nInitialize Core Data\nDatabase: Locate\nEvents: Register\nUI: Initialize\n//UI: Check Variants\n//UI: Update Controls\nUI: Update Speed/Voltage Visibility\nUI: Front Panel State >> Close", "State(s) in (\"\")"=w465) -> ("States Out"=w464:string)  [unwired: 13 in]
      }
      frame "Macro: Exit" {
        # "Exit Macro\n(This is called once, when the VI exits)"
        n209 = Unbundle By Name(w468) -> ("Core.Close Panel on Exit?"=w473:bool)
        n210 = Select(t="UI: Front Panel State >> Close", s=w473, f="") -> (s? t:f=w470:string)
        n211 = call <vilib>:"Add State(s) to Queue__JKI_lib_State_Machine.vi"("State(s) in (\"\")"=w470, "State(s) at Back (\"\")"="Data: Cleanup\nEvents: Unregister\nExit") -> ("States Out"=w467:string)  [unwired: 13 in]
        n212 = call <vilib>:"Add State(s) to Queue__JKI_lib_State_Machine.vi"("State(s) in Front (\"\")"=w467, "State(s) in (\"\")"=w476) -> ("States Out"=w475:string)  [unwired: 13 in]
      }
      frame "---------- Database ----------" {
        # "Template Separator\n(You can make a copy of, or modify, this frame)"
        n213 = call <vilib>:"Add State(s) to Queue__JKI_lib_State_Machine.vi"("State(s) in (\"\")"=w481) -> ("States Out"=w480:string)  [unwired: 14 in]
      }
      frame "Database: Set as Default" {
        # "Template Separator\n(You can make a copy of, or modify, this frame)"
        n214 = Unbundle By Name(w487) -> ("SettingDB"=w486:refnum<class "Setting Database.lvclass">)
        n215 = call "Setting Database.SetDefaultPath.vi"("error in (no error)"=w483, "SetDefaultPath"=T6 TRUE, "Setting Database"=w486) -> ("error out"=w484:errorcluster, "Setting Database out"=w485:refnum<class "Setting Database.lvclass">)  [unwired: 7 in]
        n216 = Bundle By Name(cluster=w487, "SettingDB"=w485) -> (w488:T9)
        n217 = call <vilib>:"Add State(s) to Queue__JKI_lib_State_Machine.vi"("State(s) in (\"\")"=w491) -> ("States Out"=w490:string)  [unwired: 14 in]
      }
      frame "Database: Locate" {
        w499 = refnum<class "Setting Database.lvclass"> refnum  # SettingDB
        # "#todo\nDecide what to do if not found..."
        # "Your code here.\n(You can make a copy of, or modify, this frame)"
        n218 = call <vilib>:"Create.vi"("SMO"=refnum<class "SMO.lvclass"> refnum) -> ("error out"=w495:errorcluster, "SMO out"=w505:refnum<class "SMO.lvclass">)  [unwired: 8 in, 1 out]
        n219 = call "Setting Database Name.vi"("error in (no error)"=w495) -> ("error out"=w494:errorcluster, "Name"=w502:string)  [unwired: 9 in]
        n220 = call <vilib>:"ListSharedResources.vi"("error in (no error)"=w494, "Filter (regex|name)"=w502, "SMO in"=w505) -> ("error out"=w503:errorcluster, "Shared Resources"=w501:refnum<class "SMO.lvclass">[], "SMO out"=w504:refnum<class "SMO.lvclass">)  [unwired: 5 in, 1 out]
        n221 = call <vilib>:"Destroy.vi"("error in (no error)"=w503, "SMO"=w504) -> ()  [unwired: 9 in, 1 out]
        n222 = Index Array(array=w501) -> (element=w500:refnum<class "SMO.lvclass">)  [unwired: 1 in]
        n223 = To More Specific Class(target class=w499, reference=w500) -> (specific class reference=w497:refnum<class "Setting Database.lvclass">)  [unwired: 1 in, 1 out]
        n224 = Bundle By Name(cluster=w492, "SettingDB"=w497) -> (w498:T9)
        n225 = call <vilib>:"Add State(s) to Queue__JKI_lib_State_Machine.vi"("State(s) in (\"\")"=w508) -> ("States Out"=w507:string)  [unwired: 14 in]
      }
      frame "Database: Update Active" {
        # "Your code here.\n(You can make a copy of, or modify, this frame)"
        n226 = Unbundle By Name(w514) -> ("SettingDB"=w513:refnum<class "Setting Database.lvclass">, "Path Settings"=w511:refnum<class "Path Settings.lvclass">)
        n227 = call "Setting Database.UpdateActivePath.vi"("error in (no error)"=w509, "UpdateCurrentPath"=w511, "Setting Database"=w513) -> ("error out"=w510:errorcluster, "Setting Database"=w512:refnum<class "Setting Database.lvclass">)  [unwired: 7 in]
        n228 = Bundle By Name(cluster=w514, "SettingDB"=w512) -> (w515:T9)
        n229 = call <vilib>:"Add State(s) to Queue__JKI_lib_State_Machine.vi"("State(s) in (\"\")"=w518) -> ("States Out"=w517:string)  [unwired: 14 in]
      }
      frame "Database: Copy to All" {
        # "Template Separator\n(You can make a copy of, or modify, this frame)"
        n230 = Unbundle By Name(w524) -> ("SettingDB"=w523:refnum<class "Setting Database.lvclass">)
        n231 = call "Setting Database.CopyActivePathToAll.vi"("error in (no error)"=w519, "CopyActiveToAll"=T7 TRUE, "Setting Database"=w523) -> ("error out"=w520:errorcluster, "Setting Database out"=w522:refnum<class "Setting Database.lvclass">)  [unwired: 7 in]
        n232 = Bundle By Name(cluster=w524, "SettingDB"=w522) -> (w525:T9)
        n233 = call <vilib>:"Add State(s) to Queue__JKI_lib_State_Machine.vi"("State(s) in (\"\")"=w528) -> ("States Out"=w527:string)  [unwired: 14 in]
      }
    }
  }
  n234 = disable-structure shown="Disabled" {
    frame Disabled {
      w531 = T2 {"Value"=10.0} ("Constant")
      n235 = Unbundle By Name(cluster{"Variant":variant} {"Variant"=variant}) -> ("Variant"=w530:variant)
      n236 = call <userlib>:"Get Data Name__ogtk.vi"("Data"=w531) -> ("Data Name"=w532:string)  [unwired: 8 in, 2 out]
      n237 = Get Variant Attribute(Variant=w530, name=w532, default value (empty Variant)=w531) -> ()  [unwired: 1 in, 4 out]
    }
    frame Enabled {
    }
  }
